vi "Ex_04 DataLogger.vi"(0 "VISA resource name":refnum<visa-resource-name>="COM1", 1 "baud rate":u32=9600, 2 "data bits":u16=8 min=5 max=8 step=1, 3 "parity":u16(ring) items=["None", "Odd", "Even", "Mark", "Space"], 4 "stop bits":u16(ring)=10 items=["1.0"=10, "1.5"=15, "2.0"=20], 6 "read":bool=TRUE, 7 "flow control":u16(ring) items=["None"=0, "XON/XOFF"=1, "RTS/CTS"=2, "DTR/DSR"=4]) -> (9 "read string":string, 10 "bytes read":u32)   [LabVIEW 2010]
doc: "The Basic Serial Read and Write example performs a Serial Port Read, a Serial Port Write, or a combination of these actions. The user selects the actions (read or write) on the front panel. If both are selected, the VI will write the data first, read data, and then close the VISA session that is opened to the port. This VI will wait until the specified number of bytes is received at the port. Only the number of bytes specified will be read.\n\nINSTRUCTIONS:\n1) Select the serial resource and configuration parameters (baud rate, data bits, parity, stop bits, flow control).\n2) Select the operations to be performed. \n3) Connect the serial port to your device. If no device is available, perform a loopback test by doing one of the following. Short pins 2 and 3 on a RS-232 cable or short pin 4 to pin 8 and pin 5 to pin 9 on a RS-485/422 cable. \n4) Run the VI to see the data read. (The \"read string\" will match the \"string to write\" if a loopback test was performed.)\n\nNote: The parameters set for the serial port must match the parameters of the connected instrument or device. In this example, the bytes to read parameter specifies the number of bytes that the serial port reads. If there were more bytes at the port than the number specified in bytes to read, those bytes would not be read. Also, if you specify to read more bytes than the number of bytes actually read, you might receive a timeout error message.\n\nOn the block diagram, the Configure Serial Port VI sets the configuration parameters. The front panel displays the controls used to configure the basic parameters, such as baud rate, data bits, and parity. Constants configure the other parameters the user probably does not need set. After the VISA Configure Serial Port VI opens the VISA session and configures the port, the VI passes the VISA resource name to other VIs that perform operations on that VISA resource. The VISA Write function sends a command to the serial device and the VISA Read function returns data based on the command. The VISA Close function then closes the reference to the serial device. It is important to close the reference; otherwise communication through with that port through protocols other than VISA might not be possible."
uses:
  <vilib>/Instr/_visa.llb/VISA Configure Serial Port (Instr).vi
  <vilib>/Utility/file.llb/Write To Spreadsheet File (string).vi
panel:
  in  "stop":bool
  out "Temp":dbl(graph)
  out "Temp":dbl(knob) scale=-10.0..1100.0
  in  "delay before read (ms)":u32=500
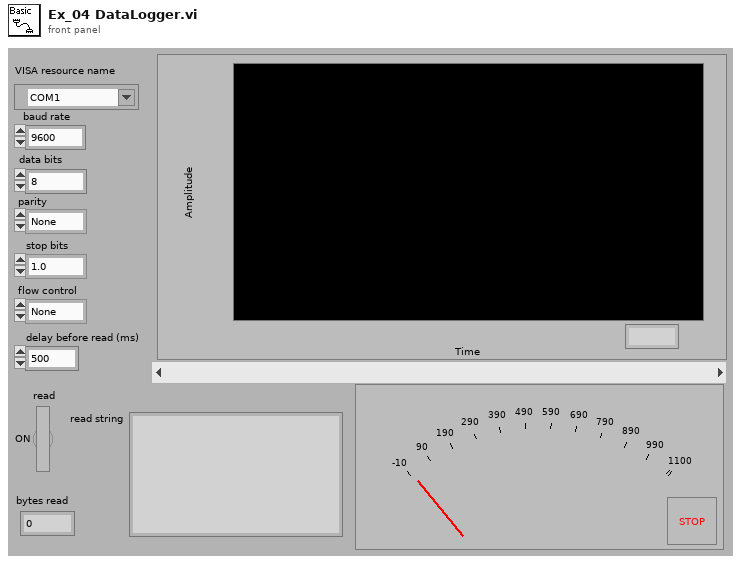
[diagram p1: front panel]
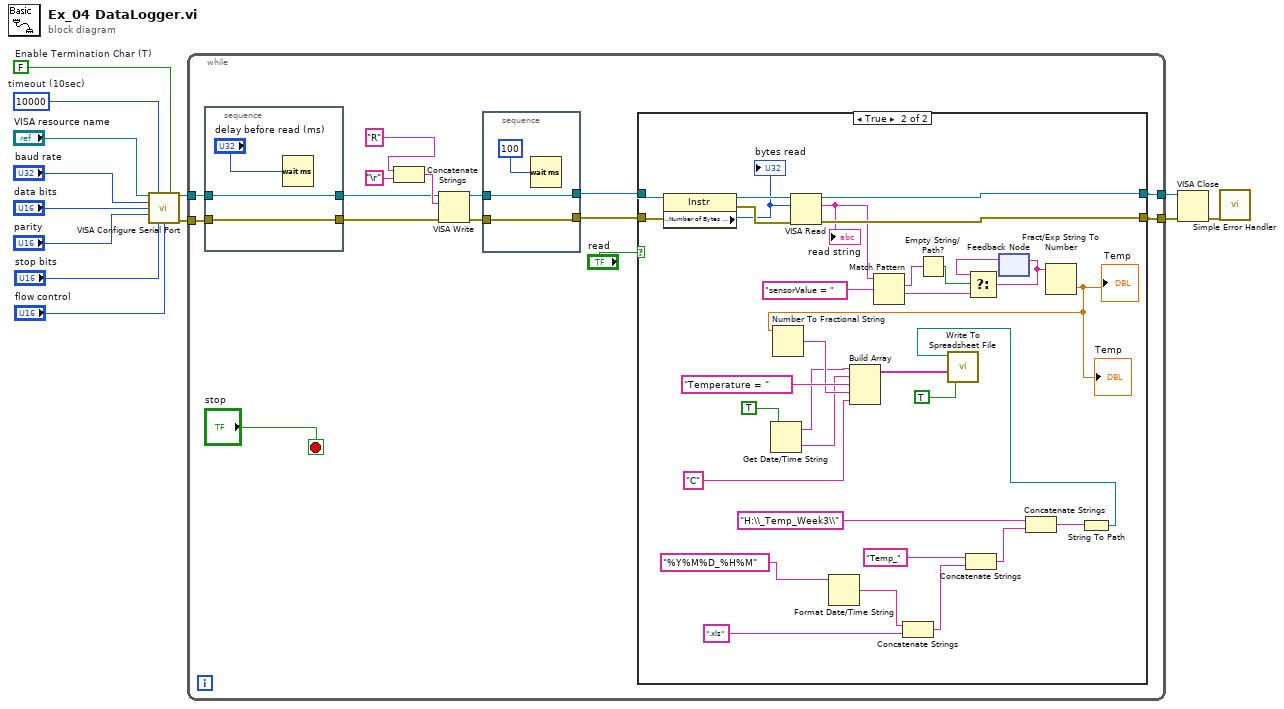
[diagram p0: block diagram]
diagram:
  w7 = FALSE  # Enable Termination Char (T)
  w8 = u32 10000  # timeout (10sec)
  n1 = call-poly "VISA Configure Serial Port"("VISA resource name"="VISA resource name", "timeout (10sec)"=w8, "Enable Termination\nChar (T)"=w7, "baud rate (9600)"="baud rate", "data bits (8)"="data bits", "parity (0:none)"="parity", "stop bits (10: 1 bit)"="stop bits", "flow control (0:none)"="flow control") -> ("VISA resource name out"=w2:refnum<visa-resource-name>, "error out"=w1:errorcluster)  [unwired: 1 in, 5 out]
  n2 = while {
    tunnel: [w27] -> w11
    tunnel: [w26] -> w3
    tunnel: w2 -> [w18]
    tunnel: w1 -> [w17]
    stop <- "stop" stop-if-true
    n3 = stacked-sequence {
      tunnel: w17 -> [w34]
      tunnel: [w34] -> w21
      tunnel: w18 -> [w33]
      tunnel: [w33] -> w22
      frame #0 {
        n4 = Wait (ms)(milliseconds to wait="delay before read (ms)") -> ()  [unwired: 1 out]
      }
    }
    n5 = Concatenate Strings("R", "\r") -> (w24:string)
    n6 = VISA Write(VISA resource name=w22, write buffer=w24, error in (no error)=w21) -> (VISA resource name out=w20:refnum<visa-resource-name>, error out=w19:errorcluster)  [unwired: 1 out]
    n7 = stacked-sequence {
      tunnel: w19 -> [w31]
      tunnel: [w31] -> w16
      tunnel: w20 -> [w30]
      tunnel: [w30] -> w15
      frame #0 {
        n8 = Wait (ms)(milliseconds to wait=u32 100 ("delay before read (ms) 2")) -> ()  [unwired: 1 out]
      }
    }
    n9 = case shown="True" "read" {
      tunnel: w16 -> [w36 w64]
      tunnel: [w36 w68] -> w26
      tunnel: [w35 w67] -> w27
      tunnel: w15 -> [w35 w66]
      frame False {
      }
      frame True {
        (unwired) "ID=13,PB1="
        n10 = property class="Instr"(reference=w66, error in=w64) -> (reference out=w65:refnum<visa-resource-name>, error out=w63:errorcluster, "Serial Settings:Number of Bytes at Serial Port"=w62:u32)
        "bytes read" <- w62
        n11 = Get Date/Time String(want seconds? (F)=TRUE) -> (date string=w47:string, time string=w46:string)  [unwired: 2 out]
        n12 = VISA Read(VISA resource name=w65, byte count=w62, error in (no error)=w63) -> (VISA resource name out=w67:refnum<visa-resource-name>, read buffer=w51:string, error out=w68:errorcluster)  [unwired: 1 out]
        "read string" <- w51
        n13 = Format Date/Time String(time format string (%c)="%Y%M%D_%H%M") -> (date/time string=w44:string)  [unwired: 2 in]
        n14 = Match Pattern(string=w51, regular expression="sensorValue = ") -> (match substring=w58:string, after substring=w57:string)  [unwired: 3 out]
        n15 = Concatenate Strings(w44, ".xls") -> (w42:string)
        n16 = Empty String/Path?(string/path=w58) -> (empty?=w60:bool)
        n17 = Concatenate Strings("Temp_", w42) -> (w39:string)
        n18 = feedback #1() -> (w59:string)  [unwired: 1 out]
        n19 = Select(t=w59, s=w60, f=w57) -> (s? t:f=w54:string)
        n20 = feedback-in #1(w54) -> ()
        n21 = Concatenate Strings("H:\\_Temp_Week3\\", w39) -> (w38:string)
        n22 = Fract/Exp String To Number(string=w54) -> (number=w50:dbl)  [unwired: 4 out]
        "Temp" <- w50
        "Temp" <- w50
        n23 = Number To Fractional String(number=w50) -> (F-format string=w52:string)  [unwired: 3 out]
        n24 = Build Array(w47, w46, "Temperature = ", w52, "C") -> (w49:string[])
        n25 = String To Path(string=w38) -> (path=w37:path)
        n26 = call-poly <vilib>:"Write To Spreadsheet File.vi"("append to file? (new file:F)"=TRUE, "1D data"=w49, "file path (dialog if empty)"=w37) -> ()  [unwired: 4 in, 2 out]
      }
    }
  }
  n27 = VISA Close(VISA resource name=w11, error in (no error)=w3) -> (error out=w10:errorcluster)
  n28 = call <vilib>:"Simple Error Handler.vi"("error in (no error)"=w10) -> ()  [unwired: 1 in, 8 out]
